vi "Write COM port.vi"(8 "error in (no error)":errorcluster, 10 "COM port":refnum<visa-resource-name>, 11 "COM Port D Element in":refnum<class "COM Port D Element.lvclass">) -> (0 "error out":errorcluster, 3 "COM Port D Element out":refnum<class "COM Port D Element.lvclass">)   [LabVIEW 2018, in "D Datagrid Library.lvlib" / "COM Port D Element.lvclass"]
uses:
  COM Port D Element.lvclass
  C:/dev/D Datagrid/String Dropdown D Element/String dropdown D Element.lvclass
  String Dropdown D Element/String dropdown D Element.lvclass/String dropdown D Element.ctl
  String Dropdown D Element/Write value.vi
  String Dropdown D Element/Write Strings.vi
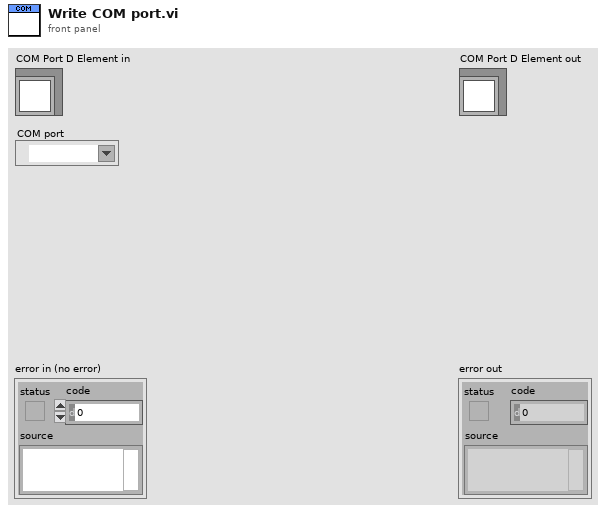
[diagram p1: front panel]
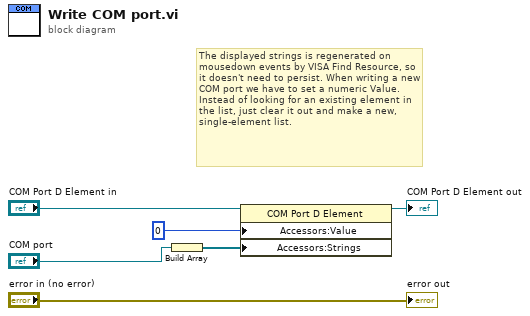
[diagram p0: block diagram]
diagram:
  # "The displayed strings is regenerated on mousedown events by VISA Find Resource, so it doesn't need to persist. When writing a new COM port we have to set a numeric Value. Instead of looking for an existing element in the list, just clear it out and make a new, single-element list."
  n1 = Build Array("COM port") -> (w2:refnum<visa-resource-name>[])
  n2 = property class="COM Port D Element"(reference="COM Port D Element in", "Accessors:Value"=0 ("Value"), "Accessors:Strings"=w2) -> (reference out=→"COM Port D Element out":refnum<class "COM Port D Element.lvclass">)  [unwired: 1 in, 1 out]
  "error out" <- "error in (no error)"
